vi "Camera Read From Laptop.vi"() -> ()   [LabVIEW 2016]
uses:
  <vilib>/Rock Robotics/WPI/Camera/WPI_CameraSettings Read MJPG.ctl
  <vilib>/Rock Robotics/WPI/Camera/WPI_CameraImageSize.ctl
  <vilib>/vision/NI_Vision_Development_Module.lvlib
panel:
  out "Veering Right":bool
  out "Error":dbl
  out "X":dbl
  out "Y":dbl
  out "Y2":dbl
  out "X2":dbl
  out "Particle Report 2":T1
  out "Particle Report":T1
  out "Bounding Box Final":T2
  in  "R/G/B":cluster{"Lower value":i32, "Upper value":i32}[](array[cluster])=[{"Lower value"=0, "Upper value"=40}, {"Lower value"=80, "Upper value"=255}, {"Lower value"=0, "Upper value"=255}]
  out "Thresholded Image":T3(plugin-control)
  in  "stop":bool
  out "error out":errorcluster
  out "Image Out":T3(plugin-control)
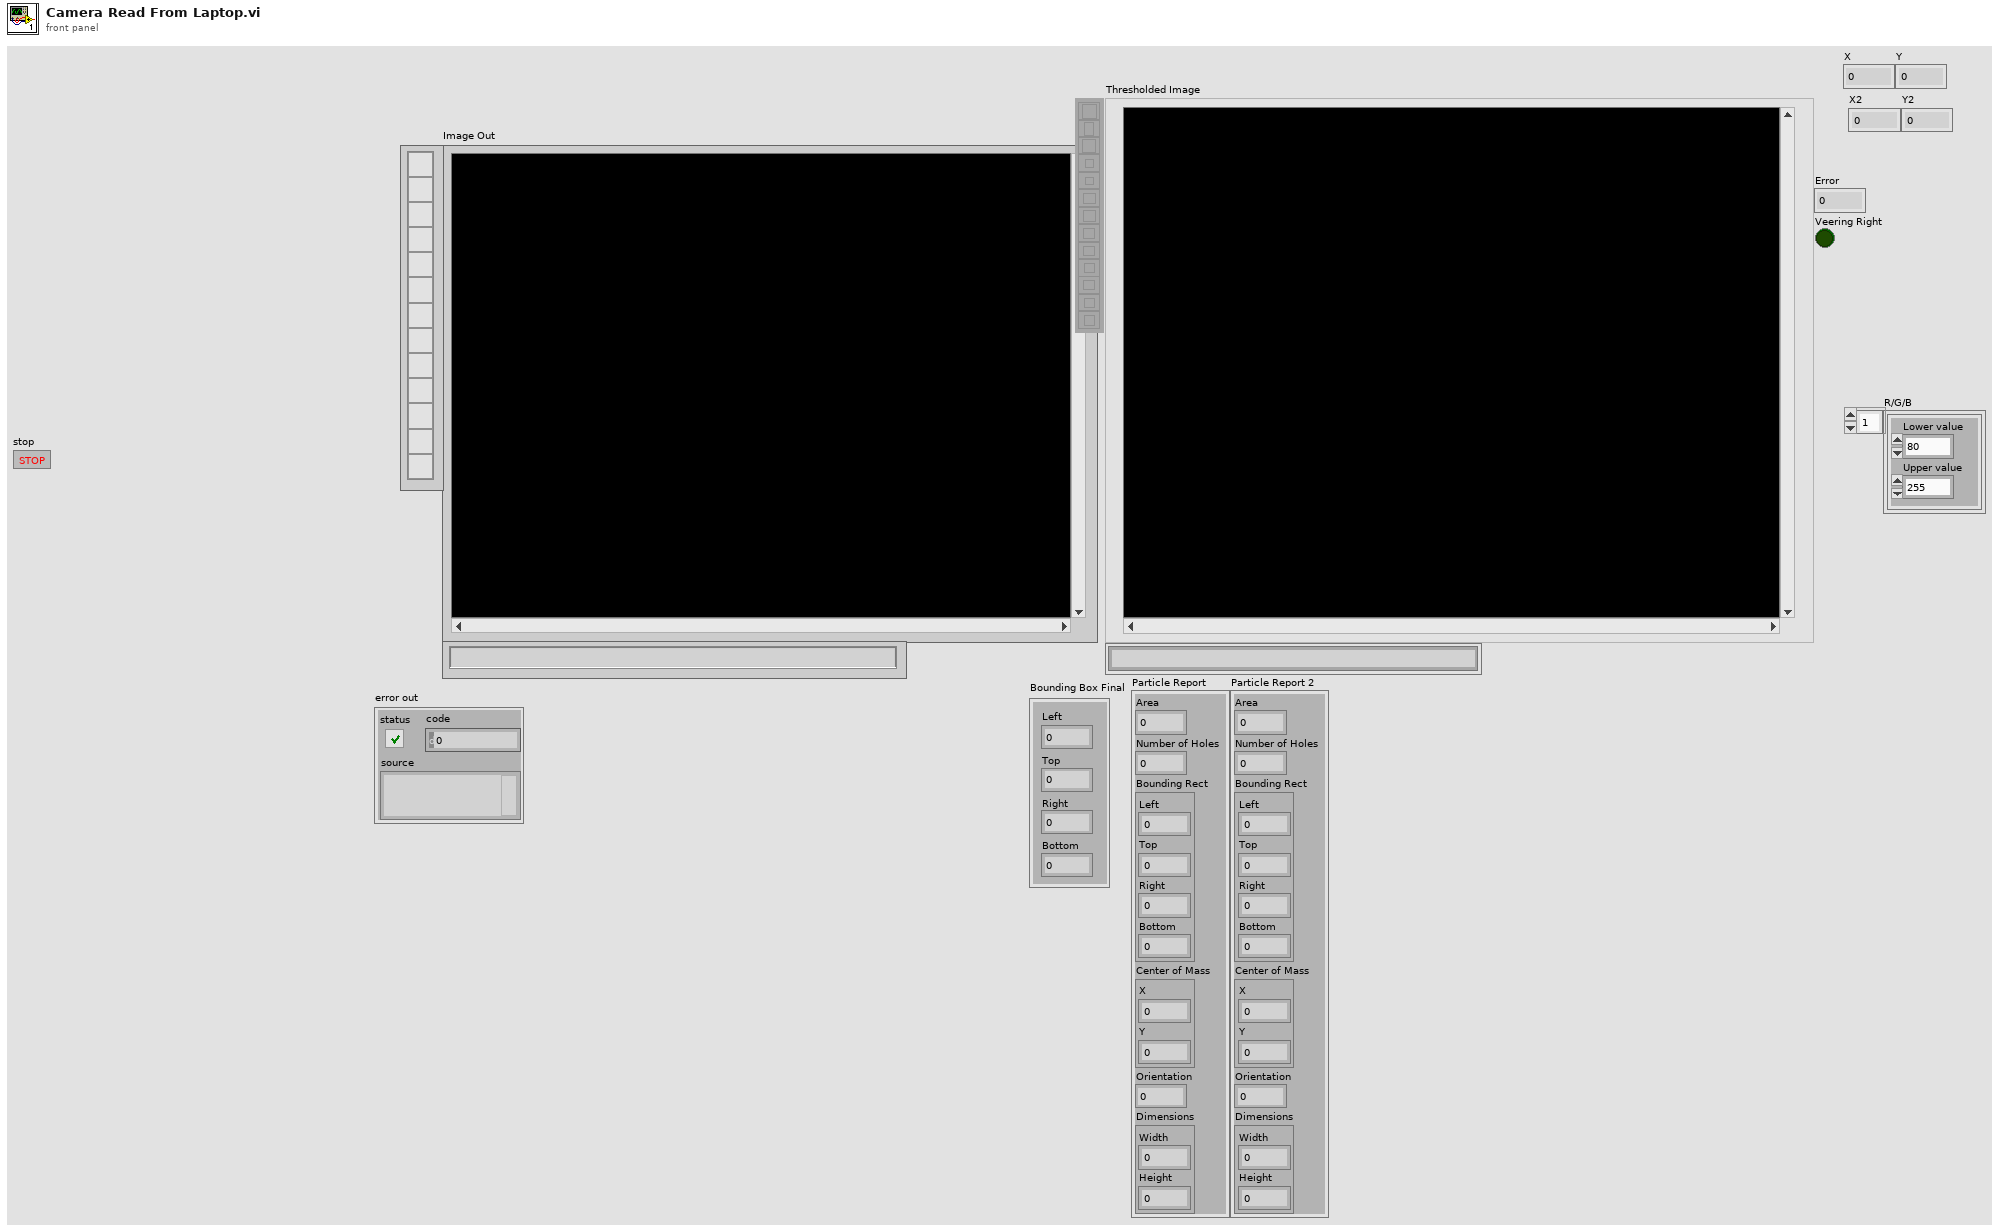
[diagram p1: front panel]
types:
  T1 = cluster{"Area":dbl, "Number of Holes":dbl, "Bounding Rect":cluster{"Left":dbl, "Top":dbl, "Right":dbl, "Bottom":dbl}, "Center of Mass":cluster{"X":dbl, "Y":dbl}, "Orientation":dbl, "Dimensions":cluster{"Width":dbl, "Height":dbl}}
  T2 = cluster{"Left":dbl, "Top":dbl, "Right":dbl, "Bottom":dbl}
  T3 = typedef "IMAQ Image.ctl" = refnum<image>
  T4 = typedef "Image Type" = u32
  T5 = typedef "WPI_CameraSettings Read MJPG.ctl" = cluster{"fps":i32, "compression":i32, "Image Size":T6, "Config Shown":bool}
  T6 = typedef "WPI_CameraImageSize.ctl" = enum16{"640x480", "320x240", "160x120", "Custom"}
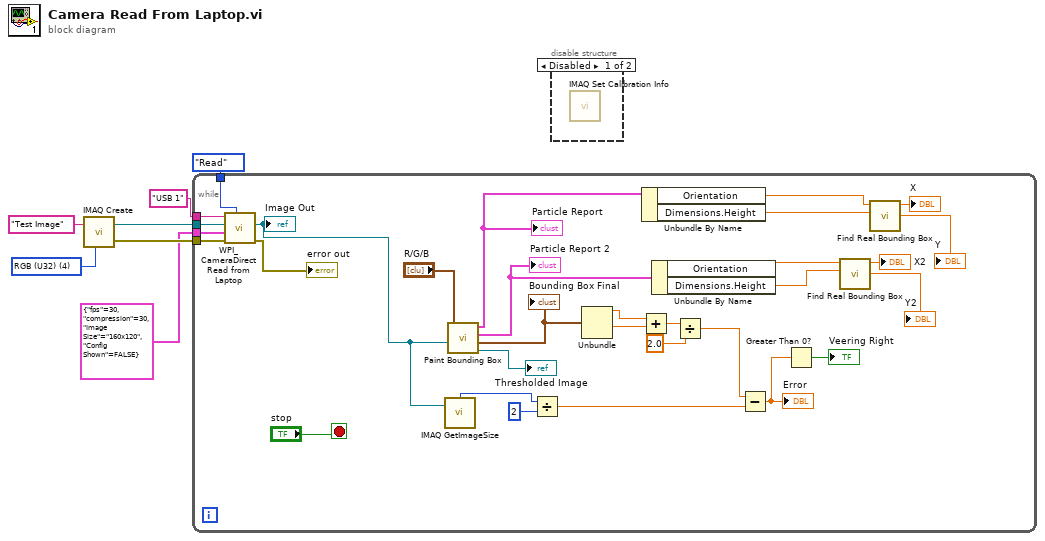
[diagram p0: block diagram]
diagram:
  w3 = T4 4 items=["Grayscale (U8)", "Grayscale (I16)", "Grayscale (SGL)", "Complex (CSG)", "RGB (U32)", "HSL (U32)", "RGB (U64)", "Grayscale (U16)"] ("Image Type")
  n1 = call "IMAQ Create"("Image Name"="Test Image", "Image Type"=w3) -> ("New Image"=w5:T3, "error out"=w6:errorcluster)  [unwired: 3 in]
  n2 = while {
    tunnel: w6 -> [w38]
    tunnel: w5 -> [w33]
    tunnel: T5 {"fps"=30, "compression"=30, "Image Size"=enum."160x120", "Config Shown"=FALSE} ("Camera Settings") -> [w37]
    tunnel: enum16{"Read", "Reopen", "Close"}."Read" ("Operation") -> [w36]
    tunnel: "USB 1" ("address") -> [w35]
    stop <- "stop" stop-if-true
    n3 = call <vilib>:"WPI_CameraDirect Read from Laptop.vi"("Operation"=w36, "error in"=w38, "Camera Settings"=w37, "Image"=w33, "address"=w35) -> ("error out"=→"error out":errorcluster, "Image Out"=w30:T3)  [unwired: 5 in]
    "Image Out" <- w30
    n4 = call "IMAQ GetImageSize"("Image"=w30) -> ("X Resolution"=w29:i32)  [unwired: 3 in, 2 out]
    n5 = call "Paint Bounding Box.vi"("Camera Image"=w30, "R/G/B"="R/G/B") -> ("Thresholded Image"=→"Thresholded Image":T3, "Bounding Box Final"=w27:T2, "Particle Report 2"=w21:T1, "Particle Report"=w14:T1)  [unwired: 5 in, 1 out]
    "Bounding Box Final" <- w27
    "Particle Report" <- w14
    "Particle Report 2" <- w21
    n6 = Divide(x=w29, y=2) -> (x/y=w10:dbl)
    n7 = Unbundle(w27) -> ("Left"=w26:dbl, "Right"=w25:dbl)  [unwired: 2 out]
    n8 = Add(x=w26, y=w25) -> (x+y=w24:dbl)
    n9 = Unbundle By Name(w14) -> ("Orientation"=w13:dbl, "Dimensions.Height"=w15:dbl)
    n10 = Unbundle By Name(w21) -> ("Orientation"=w12:dbl, "Dimensions.Height"=w20:dbl)
    n11 = Divide(x=w24, y=2.0) -> (x/y=w11:dbl)
    n12 = Subtract(x=w11, y=w10) -> (x-y=w9:dbl)
    "Error" <- w9
    n13 = Greater Than 0?(x=w9) -> (x > 0?=→"Veering Right":bool)
    n14 = call "Find Real Bounding Box.vi"("Height"=w20, "Angle"=w12) -> ("Y"=→"Y2":dbl, "X"=→"X2":dbl)  [unwired: 8 in]
    n15 = call "Find Real Bounding Box.vi"("Height"=w15, "Angle"=w13) -> ("Y"=→"Y":dbl, "X"=→"X":dbl)  [unwired: 8 in]
  }
  n16 = disable-structure shown="Disabled" {
    frame Disabled {
      n17 = call "IMAQ Set Calibration Info"() -> ()  [unwired: 10 in, 2 out]
    }
    frame Enabled {
    }
  }
